vi "Open.vi"(7 "Timeout (3000)":u32=3000, 8 "error in":errorcluster, 10 "ConfigPort (9600,0,8,1)":T1={"Baud rate"=9600, "Parity"=enum."None", "Data bits"=8, "Stop bits"=10, "Flow control"=0} {"Flow control" items=["None", "XON/XOFF", "RTS/CTS", "XON/XOFF & RTS/CTS", "DTR/DSR", "XON/XOFF & DTR/DSR"]; "Stop bits" items=["1.0"=10, "1.5"=15, "2.0"=20]}, 11 "Port(Alias)":string) -> (0 "error out":errorcluster, 1 "PortName":string, 2 "PortFound?":bool, 3 "VISA out":refnum<visa-resource-name>)   [LabVIEW 2016, in "Serial_G.lvlib"]
doc: "Open VISA"
uses:
  Serial_G.lvlib
  Controls/PortConfig.ctl
  <vilib>/Instr/_visa.llb/VISA Flush IO Buffer Mask.ctl
  <vilib>/Instr/_visa.llb/VISA Find Search Mode.ctl
  <vilib>/Utility/error.llb/Error Cluster From Error Code.vi
  <vilib>/Instr/_visa.llb/VISA Configure Serial Port (Instr).vi
  <vilib>/ErrorRing/Error Ring.xnode
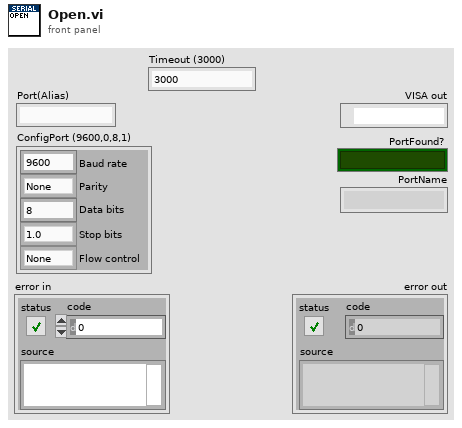
[diagram p1: front panel]
types:
  T1 = typedef "Serial_G.lvlib/PortConfig.ctl" = cluster{"Baud rate":u32, "Parity":enum16{"None", "Odd", "Even", "Mark", "Space"}, "Data bits":u16, "Stop bits":u16, "Flow control":u16}
  T2 = typedef "VISA Find Search Mode.ctl" = u32
  T3 = typedef "VISA Flush IO Buffer Mask.ctl" = u16
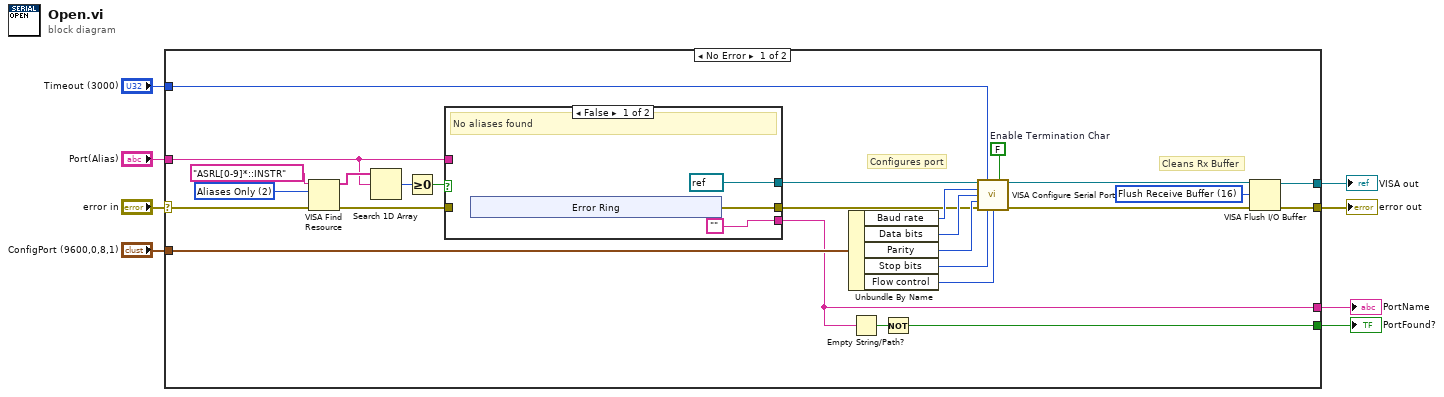
[diagram p0: block diagram]
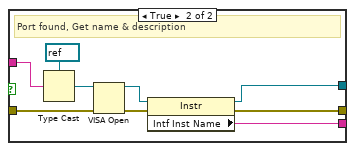
[diagram p2: hidden frame]
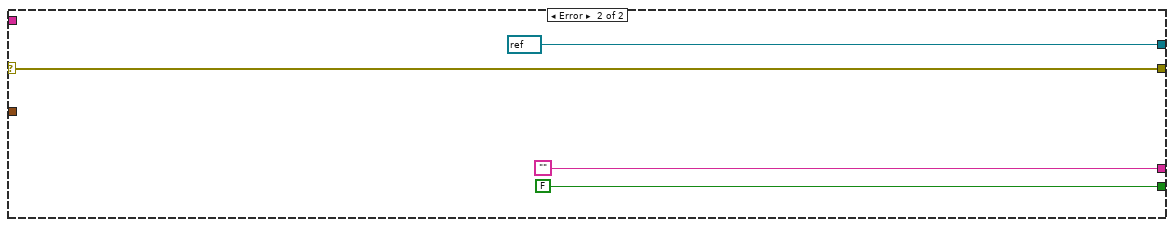
[diagram p3: hidden frame]
diagram:
  n1 = case shown="No Error" "error in" {
    selector: "error in" -> [w15 w54]
    tunnel: [w32 w54] -> w7
    tunnel: [w28 refnum<visa-resource-name> refnum ("VISA resource name out")] -> w8
    tunnel: "Timeout (3000)" -> [w13 _]
    tunnel: "ConfigPort (9600,0,8,1)" -> [w12 _]
    tunnel: "Port(Alias)" -> [w11 _]
    tunnel: [w10 "" ("Intf Inst Name")] -> w2
    tunnel: [w9 FALSE] -> w1
    frame No Error {
      w22 = T2 2 items=["Canonical Names Only"=0, "Aliases Only"=2, "Include Matching Aliases"=3, "Include All Aliases"=4] ("Search Mode")
      w33 = T3 16 items=["Flush Receive Buffer"=16, "Write Transmit Buffer to Device"=32, "Flush Receive Buffer (No I/O)"=64, "Flush Transmit Buffer"=128] ("Mask")
      w34 = FALSE  # Enable Termination Char
      # "Configures port"
      # "Cleans Rx Buffer"
      n2 = VISA Find Resource(8:w15, 10:w22, 11:"ASRL[0-9]*::INSTR" ("expression (\"?*\")")) -> (0:w17:errorcluster, 3:w18:string[])  [unwired: 1 out]
      n3 = Search 1D Array(1D array=w18, element=w11) -> (index of element=w19:i32)  [unwired: 1 in]
      n4 = Greater Or Equal To 0?(x=w19) -> (x >= 0?=w20:bool)
      n5 = case shown="False" w20 {
        tunnel: w17 -> [_ w50]
        tunnel: w11 -> [_ w46]
        tunnel: [refnum<visa-resource-name> refnum ("VISA resource name") w43] -> w16
        tunnel: [w35 w42] -> w14
        tunnel: ["" ("Intf Inst Name") w44] -> w10
        frame False {
          # "No aliases found"
          n6 = xnode "Error Ring"() -> ("error out"=w35:errorcluster)
        }
        frame True {
          # "Port found, Get name & description"
          n7 = Type Cast(type=refnum<visa-resource-name> refnum ("VISA resource name"), x=w46) -> (*(type *) &x=w45:refnum<visa-resource-name>)
          n8 = VISA Open(error in (no error)=w50, VISA resource name=w45) -> (VISA resource name=w49:refnum<visa-resource-name>, error out=w48:errorcluster)  [unwired: 3 in]
          n9 = property class="Instr"(reference=w49, error in=w48) -> (reference out=w43:refnum<visa-resource-name>, error out=w42:errorcluster, "Intf Inst Name"=w44:string)
        }
      }
      n10 = Unbundle By Name(w12) -> ("Baud rate"=w31:u32, "Data bits"=w24:u16, "Parity"=w25:enum16{"None", "Odd", "Even", "Mark", "Space"}, "Stop bits"=w30:u16, "Flow control"=w29:u16)
      n11 = Empty String/Path?(string/path=w10) -> (empty?=w23:bool)
      n12 = Not(x=w23) -> (.not. x?=w9:bool)
      n13 = call-poly "VISA Configure Serial Port"("VISA resource name"=w16, "timeout (10sec)"=w13, "Enable Termination\nChar (T)"=w34, "baud rate (9600)"=w31, "data bits (8)"=w24, "parity (0:none)"=w25, "error in (no error)"=w14, "stop bits (10: 1 bit)"=w30, "flow control (0:none)"=w29) -> ("VISA resource name out"=w27:refnum<visa-resource-name>, "error out"=w26:errorcluster)  [unwired: 5 in]
      n14 = VISA Flush I/O Buffer(VISA resource name=w27, mask (16)=w33, error in (no error)=w26) -> (VISA resource name out=w28:refnum<visa-resource-name>, error out=w32:errorcluster)
    }
    frame Error {
    }
  }
  "VISA out" <- w8
  "error out" <- w7
  "PortName" <- w2
  "PortFound?" <- w1
